vi "INIT.vi"(8 "error in (no error)":errorcluster, 11 "SIMULADO in":refnum<class "SIMULADO.lvclass">) -> (0 "error out":errorcluster, 3 "SIMULADO out":refnum<class "SIMULADO.lvclass">)   [LabVIEW 2019, in "SIMULADO.lvclass"]
uses:
  SIMULADO.lvclass
panel:
  out "read buffer 5":string
  out "read buffer 4":string
  out "read buffer 3":string
  out "read buffer 2":string
  out "read buffer":string
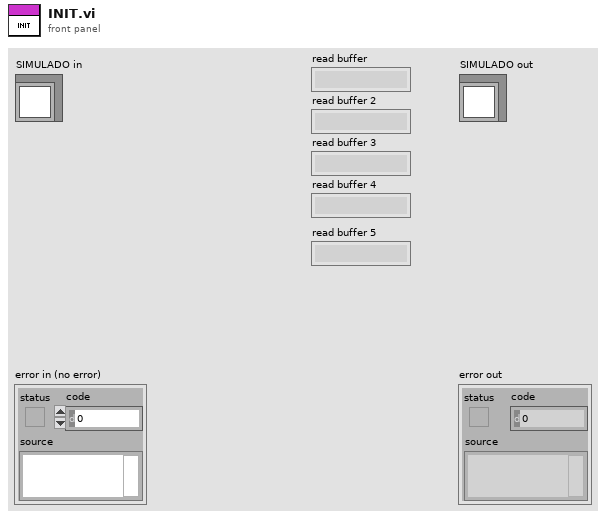
[diagram p1: front panel]
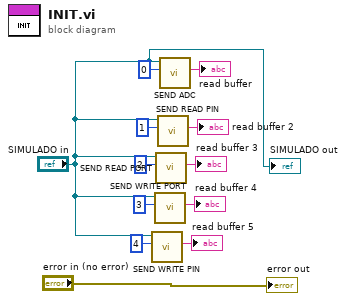
[diagram p0: block diagram]
diagram:
  n1 = call-dynamic "SEND WRITE PIN.vi"("CANAL"=u8 4, "SIMULADO in"="SIMULADO in") -> ("read buffer"=→"read buffer 5":string)  [unwired: 7 in, 2 out]
  n2 = call-dynamic "SEND WRITE PORT.vi"("CANAL"=u16 3, "SIMULADO in"="SIMULADO in") -> ("read buffer"=→"read buffer 4":string)  [unwired: 7 in, 2 out]
  n3 = call-dynamic "SEND READ PORT.vi"("CANAL"=u8 2, "SIMULADO in"="SIMULADO in") -> ("read buffer"=→"read buffer 3":string)  [unwired: 7 in, 2 out]
  n4 = call-dynamic "SEND READ PIN.vi"("CANAL"=u8 1, "SIMULADO in"="SIMULADO in") -> ("read buffer"=→"read buffer 2":string)  [unwired: 7 in, 2 out]
  n5 = call-dynamic "SEND ADC.vi"("CANAL"=u8 0, "SIMULADO in"="SIMULADO in") -> ("read buffer"=→"read buffer":string)  [unwired: 7 in, 2 out]
  "error out" <- "error in (no error)"
  "SIMULADO out" <- "SIMULADO in"
